vi "nanocal -- nuclear schottky fit -- 2x2 -- V9.vi"() -> ()   [LabVIEW 2021] (continued)
\"στS\" -> 0.003261272874   ,  \"στN\" -> 0.003231373649    |>   , \n\"IDS0512_220604_RAW_cal__sam_\" ->   <|    \"ζ\" -> 0.000000000000   ,  \"τ1\" -> 0.000000000000   ,  \"τS\" -> 0.000000000000   ,  \"τN\" -> 0.000000000000   ,  \"τC\" -> 0.000000000000   ,  \"κ0\" -> 0.000000000000   ,  \"mm1\" -> 0.000000000000   ,  \"mm2\" -> 0.000000000000   ,  \"mm3\" -> 0.000000000000   ,  \"T\" -> 0.250000000000   ,  \"B\" -> 6.000000000000   ,  \"θ\" -> 45.000000000000   ,  \"Reoff\" -> 0.000000000000   ,  \"Imoff\" -> 0.000000000000   ,  \"στ1\" -> 0.000000000000   ,  \"στS\" -> 0.000000000000   ,  \"στN\" -> 0.000000000000    |>   , \n\"IDS0513_220604_RAW_cal__ref_\" ->   <|    \"ζ\" -> 0.109354643265   ,  \"τ1\" -> 0.019745794663   ,  \"τS\" -> 0.045929868636   ,  \"τN\" -> 0.004362632792   ,  \"τC\" -> 0.001089331798   ,  \"κ0\" -> 0.000000001568   ,  \"mm1\" -> 0.000105345441   ,  \"mm2\" -> 0.017323789537   ,  \"mm3\" -> 0.059198211464   ,  \"T\" -> 0.300000000000   ,  \"B\" -> 6.000000000000   ,  \"θ\" -> 45.000000000000   ,  \"Reoff\" -> -9718367.346938773990   ,  \"Imoff\" -> 0.000000000000   ,  \"στ1\" -> 0.000746121350   ,  \"στS\" -> 0.000145078797   ,  \"στN\" -> 0.000139513521    |>   , \n\"IDS0513_220604_RAW_cal__sam_\" ->   <|    \"ζ\" -> 0.000000000000   ,  \"τ1\" -> 0.000000000000   ,  \"τS\" -> 0.000000000000   ,  \"τN\" -> 0.000000000000   ,  \"τC\" -> 0.000000000000   ,  \"κ0\" -> 0.000000000000   ,  \"mm1\" -> 0.000000000000   ,  \"mm2\" -> 0.000000000000   ,  \"mm3\" -> 0.000000000000   ,  \"T\" -> 0.300000000000   ,  \"B\" -> 6.000000000000   ,  \"θ\" -> 45.000000000000   ,  \"Reoff\" -> 0.000000000000   ,  \"Imoff\" -> 0.000000000000   ,  \"στ1\" -> 0.000000000000   ,  \"στS\" -> 0.000000000000   ,  \"στN\" -> 0.000000000000    |>   , \n\"IDS0514_220604_RAW_cal__ref_\" ->   <|    \"ζ\" -> 0.078464971050   ,  \"τ1\" -> 0.017563831776   ,  \"τS\" -> 0.042315631100   ,  \"τN\" -> 0.002449698464   ,  \"τC\" -> 0.001311085354   ,  \"κ0\" -> 0.000000001978   ,  \"mm1\" -> 0.000092908726   ,  \"mm2\" -> 0.016171593309   ,  \"mm3\" -> 0.050888254947   ,  \"T\" -> 0.360000000000   ,  \"B\" -> 6.000000000000   ,  \"θ\" -> 45.000000000000   ,  \"Reoff\" -> -5555102.040816326630   ,  \"Imoff\" -> 0.000000000000   ,  \"στ1\" -> 0.001705710692   ,  \"στS\" -> 0.000224693737   ,  \"στN\" -> 0.000168766252    |>   , \n\"IDS0514_220604_RAW_cal__sam_\" ->   <|    \"ζ\" -> 0.000000000000   ,  \"τ1\" -> 0.000000000000   ,  \"τS\" -> 0.000000000000   ,  \"τN\" -> 0.000000000000   ,  \"τC\" -> 0.000000000000   ,  \"κ0\" -> 0.000000000000   ,  \"mm1\" -> 0.000000000000   ,  \"mm2\" -> 0.000000000000   ,  \"mm3\" -> 0.000000000000   ,  \"T\" -> 0.360000000000   ,  \"B\" -> 6.000000000000   ,  \"θ\" -> 45.000000000000   ,  \"Reoff\" -> 0.000000000000   ,  \"Imoff\" -> 0.000000000000   ,  \"στ1\" -> 0.000000000000   ,  \"στS\" -> 0.000000000000   ,  \"στN\" -> 0.000000000000    |>   , \n\"IDS0515_220604_RAW_cal__ref_\" ->   <|    \"ζ\" -> 0.061585995431   ,  \"τ1\" -> 0.017021907134   ,  \"τS\" -> 0.041190711561   ,  \"τN\" -> 0.001390110365   ,  \"τC\" -> 0.001428995669   ,  \"κ0\" -> 0.000000002390   ,  \"mm1\" -> 0.000080420017   ,  \"mm2\" -> 0.016194561258   ,  \"mm3\" -> 0.047379125758   ,  \"T\" -> 0.430000000000   ,  \"B\" -> 6.000000000000   ,  \"θ\" -> 45.000000000000   ,  \"Reoff\" -> -4253061.224489795980   ,  \"Imoff\" -> 0.000000000000   ,  \"στ1\" -> 0.004152949973   ,  \"στS\" -> 0.000363204682   ,  \"στN\" -> 0.000192260687    |>   , \n\"IDS0515_220604_RAW_cal__sam_\" ->   <|    \"ζ\" -> 0.000000000000   ,  \"τ1\" -> 0.000000000000   ,  \"τS\" -> 0.000000000000   ,  \"τN\" -> 0.000000000000   ,  \"τC\" -> 0.000000000000   ,  \"κ0\" -> 0.000000000000   ,  \"mm1\" -> 0.000000000000   ,  \"mm2\" -> 0.000000000000   ,  \"mm3\" -> 0.000000000000   ,  \"T\" -> 0.430000000000   ,  \"B\" -> 6.000000000000   ,  \"θ\" -> 45.000000000000   ,  \"Reoff\" -> 0.000000000000   ,  \"Imoff\" -> 0.000000000000   ,  \"στ1\" -> 0.000000000000   ,  \"στS\" -> 0.000000000000   ,  \"στN\" -> 0.000000000000    |>   , \n\"IDS0516_220604_RAW_cal__ref_\" ->   <|    \"ζ\" -> 0.045061124228   ,  \"τ1\" -> 0.016174333666   ,  \"τS\" -> 0.041331628225   ,  \"τN\" -> 0.001008746985   ,  \"τC\" -> 0.001666143406   ,  \"κ0\" -> 0.000000003072   ,  \"mm1\" -> 0.000069279556   ,  \"mm2\" -> 0.015610467629   ,  \"mm3\" -> 0.046409010004   ,  \"T\" -> 0.520000000000   ,  \"B\" -> 6.000000000000   ,  \"θ\" -> 45.000000000000   ,  \"Reoff\" -> -2636734.693877550770   ,  \"Imoff\" -> 0.000000000000   ,  \"στ1\" -> 0.000679845630   ,  \"στS\" -> 0.000215440983   ,  \"στN\" -> 0.000036761910    |>   , \n\"IDS0516_220604_RAW_cal__sam_\" ->   <|    \"ζ\" -> 0.000000000000   ,  \"τ1\" -> 0.000000000000   ,  \"τS\" -> 0.000000000000   ,  \"τN\" -> 0.000000000000   ,  \"τC\" -> 0.000000000000   ,  \"κ0\" -> 0.000000000000   ,  \"mm1\" -> 0.000000000000   ,  \"mm2\" -> 0.000000000000   ,  \"mm3\" -> 0.000000000000   ,  \"T\" -> 0.520000000000   ,  \"B\" -> 6.000000000000   ,  \"θ\" -> 45.000000000000   ,  \"Reoff\" -> 0.000000000000   ,  \"Imoff\" -> 0.000000000000   ,  \"στ1\" -> 0.000000000000   ,  \"στS\" -> 0.000000000000   ,  \"στN\" -> 0.000000000000    |>   , \n\"IDS0517_220604_RAW_cal__ref_\" ->   <|    \"ζ\" -> 0.037661249073   ,  \"τ1\" -> 0.016158267438   ,  \"τS\" -> 0.041535470501   ,  \"τN\" -> 0.000589951470   ,  \"τC\" -> 0.001574909889   ,  \"κ0\" -> 0.000000003727   ,  \"mm1\" -> 0.000055213424   ,  \"mm2\" -> 0.015821969361   ,  \"mm3\" -> 0.045567912522   ,  \"T\" -> 0.620000000000   ,  \"B\" -> 6.000000000000   ,  \"θ\" -> 45.000000000000   ,  \"Reoff\" -> -2277551.020408163780   ,  \"Imoff\" -> 0.000000000000   ,  \"στ1\" -> 0.000926762360   ,  \"στS\" -> 0.000192613038   ,  \"στN\" -> 0.000026616394    |>   , \n\"IDS0517_220604_RAW_cal__sam_\" ->   <|    \"ζ\" -> 0.000000000000   ,  \"τ1\" -> 0.000000000000   ,  \"τS\" -> 0.000000000000   ,  \"τN\" -> 0.000000000000   ,  \"τC\" -> 0.000000000000   ,  \"κ0\" -> 0.000000000000   ,  \"mm1\" -> 0.000000000000   ,  \"mm2\" -> 0.000000000000   ,  \"mm3\" -> 0.000000000000   ,  \"T\" -> 0.620000000000   ,  \"B\" -> 6.000000000000   ,  \"θ\" -> 45.000000000000   ,  \"Reoff\" -> 0.000000000000   ,  \"Imoff\" -> 0.000000000000   ,  \"στ1\" -> 0.000000000000   ,  \"στS\" -> 0.000000000000   ,  \"στN\" -> 0.000000000000    |>   , \n\"IDS0518_220604_RAW_cal__ref_\" ->   <|    \"ζ\" -> 0.026897195586   ,  \"τ1\" -> 0.017029322947   ,  \"τS\" -> 0.030300618121   ,  \"τN\" -> 0.000253092893   ,  \"τC\" -> 0.002128020527   ,  \"κ0\" -> 0.000000005137   ,  \"mm1\" -> 0.000052252635   ,  \"mm2\" -> 0.016764147571   ,  \"mm3\" -> 0.033716463424   ,  \"T\" -> 0.820000000000   ,  \"B\" -> 6.000000000000   ,  \"θ\" -> 45.000000000000   ,  \"Reoff\" -> -1020408.163265306500   ,  \"Imoff\" -> 0.000000000000   ,  \"στ1\" -> 0.001120431630   ,  \"στS\" -> 0.000175631796   ,  \"στN\" -> 0.000008557959    |>   , \n\"IDS0518_220604_RAW_cal__sam_\" ->   <|    \"ζ\" -> 0.000000000000   ,  \"τ1\" -> 0.000000000000   ,  \"τS\" -> 0.000000000000   ,  \"τN\" -> 0.000000000000   ,  \"τC\" -> 0.000000000000   ,  \"κ0\" -> 0.000000000000   ,  \"mm1\" -> 0.000000000000   ,  \"mm2\" -> 0.000000000000   ,  \"mm3\" -> 0.000000000000   ,  \"T\" -> 0.820000000000   ,  \"B\" -> 6.000000000000   ,  \"θ\" -> 45.000000000000   ,  \"Reoff\" -> 0.000000000000   ,  \"Imoff\" -> 0.000000000000   ,  \"στ1\" -> 0.000000000000   ,  \"στS\" -> 0.000000000000   ,  \"στN\" -> 0.000000000000    |>   , \n\"IDS0519_220604_RAW_cal__ref_\" ->   <|    \"ζ\" -> 0.022664825895   ,  \"τ1\" -> 0.014721420139   ,  \"τS\" -> 0.018200510248   ,  \"τN\" -> 0.000100851172   ,  \"τC\" -> 0.002380537737   ,  \"κ0\" -> 0.000000007190   ,  \"mm1\" -> 0.000046880798   ,  \"mm2\" -> 0.014490052902   ,  \"mm3\" -> 0.021281182766   ,  \"T\" -> 1.120000000000   ,  \"B\" -> 6.000000000000   ,  \"θ\" -> 45.000000000000   ,  \"Reoff\" -> -795918.367346938698   ,  \"Imoff\" -> 0.000000000000   ,  \"στ1\" -> 0.002006498411   ,  \"στS\" -> 0.000156945460   ,  \"στN\" -> 0.000006591622    |>   , \n\"IDS0519_220604_RAW_cal__sam_\" ->   <|    \"ζ\" -> 0.000000000000   ,  \"τ1\" -> 0.000000000000   ,  \"τS\" -> 0.000000000000   ,  \"τN\" -> 0.000000000000   ,  \"τC\" -> 0.000000000000   ,  \"κ0\" -> 0.000000000000   ,  \"mm1\" -> 0.000000000000   ,  \"mm2\" -> 0.000000000000   ,  \"mm3\" -> 0.000000000000   ,  \"T\" -> 1.120000000000   ,  \"B\" -> 6.000000000000   ,  \"θ\" -> 45.000000000000   ,  \"Reoff\" -> 0.000000000000   ,  \"Imoff\" -> 0.000000000000   ,  \"στ1\" -> 0.000000000000   ,  \"στS\" -> 0.000000000000   ,  \"στN\" -> 0.000000000000    |>   , \n\"IDS0520_220604_RAW_cal__ref_\" ->   <|    \"ζ\" -> 0.017334133227   ,  \"τ1\" -> 0.014742496640   ,  \"τS\" -> 0.012814930706   ,  \"τN\" -> 0.000029321869   ,  \"τC\" -> 0.002644067199   ,  \"κ0\" -> 0.000000012608   ,  \"mm1\" -> 0.000037545170   ,  \"mm2\" -> 0.014397895803   ,  \"mm3\" -> 0.016018019426   ,  \"T\" -> 1.900000000000   ,  \"B\" -> 6.000000000000   ,  \"θ\" -> 45.000000000000   ,  \"Reoff\" -> -346938.775510204955   ,  \"Imoff\" -> 0.000000000000   ,  \"στ1\" -> 0.000944080066   ,  \"στS\" -> 0.000100682155   ,  \"στN\" -> 0.000000473993    |>   , \n\"IDS0520_220604_RAW_cal__sam_\" ->   <|    \"ζ\" -> 0.000000000000   ,  \"τ1\" -> 0.000000000000   ,  \"τS\" -> 0.000000000000   ,  \"τN\" -> 0.000000000000   ,  \"τC\" -> 0.000000000000   ,  \"κ0\" -> 0.000000000000   ,  \"mm1\" -> 0.000000000000   ,  \"mm2\" -> 0.000000000000   ,  \"mm3\" -> 0.000000000000   ,  \"T\" -> 1.900000000000   ,  \"B\" -> 6.000000000000   ,  \"θ\" -> 45.000000000000   ,  \"Reoff\" -> 0.000000000000   ,  \"Imoff\" -> 0.000000000000   ,  \"στ1\" -> 0.000000000000   ,  \"στS\" -> 0.000000000000   ,  \"στN\" -> 0.000000000000    |>   , \n\"IDS0521_220604_RAW_cal__ref_\" ->   <|    \"ζ\" -> 0.016488778700   ,  \"τ1\" -> 0.014739187925   ,  \"τS\" -> 0.009276506923   ,  \"τN\" -> 0.000009013062   ,  \"τC\" -> 0.002584186338   ,  \"κ0\" -> 0.000000022490   ,  \"mm1\" -> 0.000032992550   ,  \"mm2\" -> 0.011941581665   ,  \"mm3\" -> 0.014787426917   ,  \"T\" -> 3.100000000000   ,  \"B\" -> 6.000000000000   ,  \"θ\" -> 45.000000000000   ,  \"Reoff\" -> -167346.938775509596   ,  \"Imoff\" -> 0.000000000000   ,  \"στ1\" -> 0.000306328571   ,  \"στS\" -> 0.000088607277   ,  \"στN\" -> 0.000000155207    |>   , \n\"IDS0521_220604_RAW_cal__sam_\" ->   <|    \"ζ\" -> 0.000000000000   ,  \"τ1\" -> 0.000000000000   ,  \"τS\" -> 0.000000000000   ,  \"τN\" -> 0.000000000000   ,  \"τC\" -> 0.000000000000   ,  \"κ0\" -> 0.000000000000   ,  \"mm1\" -> 0.000000000000   ,  \"mm2\" -> 0.000000000000   ,  \"mm3\" -> 0.000000000000   ,  \"T\" -> 3.100000000000   ,  \"B\" -> 6.000000000000   ,  \"θ\" -> 45.000000000000   ,  \"Reoff\" -> 0.000000000000   ,  \"Imoff\" -> 0.000000000000   ,  \"στ1\" -> 0.000000000000   ,  \"στS\" -> 0.000000000000   ,  \"στN\" -> 0.000000000000    |>   , \n\"IDS0523_220604_RAW_cal__ref_\" ->   <|    \"ζ\" -> 0.248494287035   ,  \"τ1\" -> 0.140471463831   ,  \"τS\" -> 0.029170563772   ,  \"τN\" -> 0.016077523258   ,  \"τC\" -> 0.000858124054   ,  \"κ0\" -> 0.000000000897   ,  \"mm1\" -> 0.000167616779   ,  \"mm2\" -> 0.031344824749   ,  \"mm3\" -> 0.166309124513   ,  \"T\" -> 0.200000000000   ,  \"B\" -> 4.000000000000   ,  \"θ\" -> 45.000000000000   ,  \"Reoff\" -> -41942857.142857194000   ,  \"Imoff\" -> 0.000000000000   ,  \"στ1\" -> 0.163113161678   ,  \"στS\" -> 0.000492211177   ,  \"στN\" -> 0.015881366148    |>   , \n\"IDS0523_220604_RAW_cal__sam_\" ->   <|    \"ζ\" -> 0.000000000000   ,  \"τ1\" -> 0.000000000000   ,  \"τS\" -> 0.000000000000   ,  \"τN\" -> 0.000000000000   ,  \"τC\" -> 0.000000000000   ,  \"κ0\" -> 0.000000000000   ,  \"mm1\" -> 0.000000000000   ,  \"mm2\" -> 0.000000000000   ,  \"mm3\" -> 0.000000000000   ,  \"T\" -> 0.200000000000   ,  \"B\" -> 4.000000000000   ,  \"θ\" -> 45.000000000000   ,  \"Reoff\" -> 0.000000000000   ,  \"Imoff\" -> 0.000000000000   ,  \"στ1\" -> 0.000000000000   ,  \"στS\" -> 0.000000000000   ,  \"στN\" -> 0.000000000000    |>   , \n\"IDS0524_220605_RAW_cal__ref_\" ->   <|    \"ζ\" -> 0.342264426031   ,  \"τ1\" -> 0.148951865550   ,  \"τS\" -> 0.034223286872   ,  \"τN\" -> 0.023114154081   ,  \"τC\" -> 0.000835537193   ,  \"κ0\" -> 0.000000000715   ,  \"mm1\" -> 0.000210189792   ,  \"mm2\" -> 0.036494538053   ,  \"mm3\" -> 0.190044682168   ,  \"T\" -> 0.170000000000   ,  \"B\" -> 4.000000000000   ,  \"θ\" -> 45.000000000000   ,  \"Reoff\" -> -68526530.612244904100   ,  \"Imoff\" -> 0.000000000000   ,  \"στ1\" -> 0.142355896146   ,  \"στS\" -> 0.002021018584   ,  \"στN\" -> 0.017181504971    |>   , \n\"IDS0524_220605_RAW_cal__sam_\" ->   <|    \"ζ\" -> 0.000000000000   ,  \"τ1\" -> 0.000000000000   ,  \"τS\" -> 0.000000000000   ,  \"τN\" -> 0.000000000000   ,  \"τC\" -> 0.000000000000   ,  \"κ0\" -> 0.000000000000   ,  \"mm1\" -> 0.000000000000   ,  \"mm2\" -> 0.000000000000   ,  \"mm3\" -> 0.000000000000   ,  \"T\" -> 0.170000000000   ,  \"B\" -> 4.000000000000   ,  \"θ\" -> 45.000000000000   ,  \"Reoff\" -> 0.000000000000   ,  \"Imoff\" -> 0.000000000000   ,  \"στ1\" -> 0.000000000000   ,  \"στS\" -> 0.000000000000   ,  \"στN\" -> 0.000000000000    |>   , \n\"IDS0525_220605_RAW_cal__ref_\" ->   <|    \"ζ\" -> 0.438280595131   ,  \"τ1\" -> 0.137342772879   ,  \"τS\" -> 0.040264580872   ,  \"τN\" -> 0.033372414925   ,  \"τC\" -> 0.000857425660   ,  \"κ0\" -> 0.000000000589   ,  \"mm1\" -> 0.000258601158   ,  \"mm2\" -> 0.039283249404   ,  \"mm3\" -> 0.204569010116   ,  \"T\" -> 0.150000000000   ,  \"B\" -> 4.000000000000   ,  \"θ\" -> 45.000000000000   ,  \"Reoff\" -> -86930612.244897961600   ,  \"Imoff\" -> 0.000000000000   ,  \"στ1\" -> 0.199442289109   ,  \"στS\" -> 0.005269413629   ,  \"στN\" -> 0.036619051524    |>   , \n\"IDS0525_220605_RAW_cal__sam_\" ->   <|    \"ζ\" -> 0.000000000000   ,  \"τ1\" -> 0.000000000000   ,  \"τS\" -> 0.000000000000   ,  \"τN\" -> 0.000000000000   ,  \"τC\" -> 0.000000000000   ,  \"κ0\" -> 0.000000000000   ,  \"mm1\" -> 0.000000000000   ,  \"mm2\" -> 0.000000000000   ,  \"mm3\" -> 0.000000000000   ,  \"T\" -> 0.150000000000   ,  \"B\" -> 4.000000000000   ,  \"θ\" -> 45.000000000000   ,  \"Reoff\" -> 0.000000000000   ,  \"Imoff\" -> 0.000000000000   ,  \"στ1\" -> 0.000000000000   ,  \"στS\" -> 0.000000000000   ,  \"στN\" -> 0.000000000000    |>   , \n\"IDS0526_220605_RAW_cal__ref_\" ->   <|    \"ζ\" -> 0.681535842582   ,  \"τ1\" -> 0.096440830636   ,  \"τS\" -> 0.049346041453   ,  \"τN\" -> 0.056139024949   ,  \"τC\" -> 0.000822867948   ,  \"κ0\" -> 0.000000000444   ,  \"mm1\" -> 0.000331542094   ,  \"mm2\" -> 0.033417308945   ,  \"mm3\" -> 0.240891767557   ,  \"T\" -> 0.120000000000   ,  \"B\" -> 4.000000000000   ,  \"θ\" -> 45.000000000000   ,  \"Reoff\" -> -183040816.326530635000   ,  \"Imoff\" -> 0.000000000000   ,  \"στ1\" -> 0.106020317496   ,  \"στS\" -> 0.010756317478   ,  \"στN\" -> 0.041433473525    |>   , \n\"IDS0526_220605_RAW_cal__sam_\" ->   <|    \"ζ\" -> 0.000000000000   ,  \"τ1\" -> 0.000000000000   ,  \"τS\" -> 0.000000000000   ,  \"τN\" -> 0.000000000000   ,  \"τC\" -> 0.000000000000   ,  \"κ0\" -> 0.000000000000   ,  \"mm1\" -> 0.000000000000   ,  \"mm2\" -> 0.000000000000   ,  \"mm3\" -> 0.000000000000   ,  \"T\" -> 0.120000000000   ,  \"B\" -> 4.000000000000   ,  \"θ\" -> 45.000000000000   ,  \"Reoff\" -> 0.000000000000   ,  \"Imoff\" -> 0.000000000000   ,  \"στ1\" -> 0.000000000000   ,  \"στS\" -> 0.000000000000   ,  \"στN\" -> 0.000000000000    |>   , \n\"IDS0527_220605_RAW_cal__ref_\" ->   <|    \"ζ\" -> 0.163587274330   ,  \"τ1\" -> 0.177723598175   ,  \"τS\" -> 0.024747362505   ,  \"τN\" -> 0.010499593471   ,  \"τC\" -> 0.000964995814   ,  \"κ0\" -> 0.000000001207   ,  \"mm1\" -> 0.000131851499   ,  \"mm2\" -> 0.027402099160   ,  \"mm3\" -> 0.192167552763   ,  \"T\" -> 0.250000000000   ,  \"B\" -> 4.000000000000   ,  \"θ\" -> 45.000000000000   ,  \"Reoff\" -> -21493877.551020443400   ,  \"Imoff\" -> 0.000000000000   ,  \"στ1\" -> 0.096620218228   ,  \"στS\" -> 0.000434999932   ,  \"στN\" -> 0.007322093866    |>   , \n\"IDS0527_220605_RAW_cal__sam_\" ->   <|    \"ζ\" -> 0.000000000000   ,  \"τ1\" -> 0.000000000000   ,  \"τS\" -> 0.000000000000   ,  \"τN\" -> 0.000000000000   ,  \"τC\" -> 0.000000000000   ,  \"κ0\" -> 0.000000000000   ,  \"mm1\" -> 0.000000000000   ,  \"mm2\" -> 0.000000000000   ,  \"mm3\" -> 0.000000000000   ,  \"T\" -> 0.250000000000   ,  \"B\" -> 4.000000000000   ,  \"θ\" -> 45.000000000000   ,  \"Reoff\" -> 0.000000000000   ,  \"Imoff\" -> 0.000000000000   ,  \"στ1\" -> 0.000000000000   ,  \"στS\" -> 0.000000000000   ,  \"στN\" -> 0.000000000000    |>   , \n\"IDS0528_220605_RAW_cal__ref_\" ->   <|    \"ζ\" -> 0.115342924881   ,  \"τ1\" -> 0.183028972039   ,  \"τS\" -> 0.022615118092   ,  \"τN\" -> 0.006941794186   ,  \"τC\" -> 0.001037906865   ,  \"κ0\" -> 0.000000001545   ,  \"mm1\" -> 0.000103500075   ,  \"mm2\" -> 0.024936932480   ,  \"mm3\" -> 0.191992539340   ,  \"T\" -> 0.300000000000   ,  \"B\" -> 4.000000000000   ,  \"θ\" -> 45.000000000000   ,  \"Reoff\" -> -13363265.306122444600   ,  \"Imoff\" -> 0.000000000000   ,  \"στ1\" -> 0.063499413801   ,  \"στS\" -> 0.000291757985   ,  \"στN\" -> 0.002527808179    |>   , \n\"IDS0528_220605_RAW_cal__sam_\" ->   <|    \"ζ\" -> 0.000000000000   ,  \"τ1\" -> 0.000000000000   ,  \"τS\" -> 0.000000000000   ,  \"τN\" -> 0.000000000000   ,  \"τC\" -> 0.000000000000   ,  \"κ0\" -> 0.000000000000   ,  \"mm1\" -> 0.000000000000   ,  \"mm2\" -> 0.000000000000   ,  \"mm3\" -> 0.000000000000   ,  \"T\" -> 0.300000000000   ,  \"B\" -> 4.000000000000   ,  \"θ\" -> 45.000000000000   ,  \"Reoff\" -> 0.000000000000   ,  \"Imoff\" -> 0.000000000000   ,  \"στ1\" -> 0.000000000000   ,  \"στS\" -> 0.000000000000   ,  \"στN\" -> 0.000000000000    |>   , \n\"IDS0529_220605_RAW_cal__ref_\" ->   <|    \"ζ\" -> 0.082205302754   ,  \"τ1\" -> 0.199068291340   ,  \"τS\" -> 0.021395603563   ,  \"τN\" -> 0.004747138238   ,  \"τC\" -> 0.001295613399   ,  \"κ0\" -> 0.000000001948   ,  \"mm1\" -> 0.000093558415   ,  \"mm2\" -> 0.023663557896   ,  \"mm3\" -> 0.204898602234   ,  \"T\" -> 0.360000000000   ,  \"B\" -> 4.000000000000   ,  \"θ\" -> 45.000000000000   ,  \"Reoff\" -> -6702040.816326528790   ,  \"Imoff\" -> 0.000000000000   ,  \"στ1\" -> 0.038070369381   ,  \"στS\" -> 0.000151057018   ,  \"στN\" -> 0.001245904687    |>   , \n\"IDS0529_220605_RAW_cal__sam_\" ->   <|    \"ζ\" -> 0.000000000000   ,  \"τ1\" -> 0.000000000000   ,  \"τS\" -> 0.000000000000   ,  \"τN\" -> 0.000000000000   ,  \"τC\" -> 0.000000000000   ,  \"κ0\" -> 0.000000000000   ,  \"mm1\" -> 0.000000000000   ,  \"mm2\" -> 0.000000000000   ,  \"mm3\" -> 0.000000000000   ,  \"T\" -> 0.360000000000   ,  \"B\" -> 4.000000000000   ,  \"θ\" -> 45.000000000000   ,  \"Reoff\" -> 0.000000000000   ,  \"Imoff\" -> 0.000000000000   ,  \"στ1\" -> 0.000000000000   ,  \"στS\" -> 0.000000000000   ,  \"στN\" -> 0.000000000000    |>   , \n\"IDS0530_220605_RAW_cal__ref_\" ->   <|    \"ζ\" -> 0.062434773086   ,  \"τ1\" -> 0.091033034747   ,  \"τS\" -> 0.021000801063   ,  \"τN\" -> 0.002166413652   ,  \"τC\" -> 0.001607646673   ,  \"κ0\" -> 0.000000002334   ,  \"mm1\" -> 0.000088451406   ,  \"mm2\" -> 0.023050943702   ,  \"mm3\" -> 0.094114940821   ,  \"T\" -> 0.420000000000   ,  \"B\" -> 4.000000000000   ,  \"θ\" -> 45.000000000000   ,  \"Reoff\" -> -3579591.836734689770   ,  \"Imoff\" -> 0.000000000000   ,  \"στ1\" -> 0.001625101640   ,  \"στS\" -> 0.000103039832   ,  \"στN\" -> 0.000006624579    |>   , \n\"IDS0530_220605_RAW_cal__sam_\" ->   <|    \"ζ\" -> 0.000000000000   ,  \"τ1\" -> 0.000000000000   ,  \"τS\" -> 0.000000000000   ,  \"τN\" -> 0.000000000000   ,  \"τC\" -> 0.000000000000   ,  \"κ0\" -> 0.000000000000   ,  \"mm1\" -> 0.000000000000   ,  \"mm2\" -> 0.000000000000   ,  \"mm3\" -> 0.000000000000   ,  \"T\" -> 0.420000000000   ,  \"B\" -> 4.000000000000   ,  \"θ\" -> 45.000000000000   ,  \"Reoff\" -> 0.000000000000   ,  \"Imoff\" -> 0.000000000000   ,  \"στ1\" -> 0.000000000000   ,  \"στS\" -> 0.000000000000   ,  \"στN\" -> 0.000000000000    |>   , \n\"IDS0531_220605_RAW_cal__ref_\" ->   <|    \"ζ\" -> 0.047292360430   ,  \"τ1\" -> 0.215650832524   ,  \"τS\" -> 0.021748628873   ,  \"τN\" -> 0.002014257649   ,  \"τC\" -> 0.001656178311   ,  \"κ0\" -> 0.000000003034   ,  \"mm1\" -> 0.000069918264   ,  \"mm2\" -> 0.024098100915   ,  \"mm3\" -> 0.218025681173   ,  \"T\" -> 0.520000000000   ,  \"B\" -> 4.000000000000   ,  \"θ\" -> 45.000000000000   ,  \"Reoff\" -> -2955102.040816321970   ,  \"Imoff\" -> 0.000000000000   ,  \"στ1\" -> 0.046963197390   ,  \"στS\" -> 0.000145543572   ,  \"στN\" -> 0.000181922698    |>   , \n\"IDS0531_220605_RAW_cal__sam_\" ->   <|    \"ζ\" -> 0.000000000000   ,  \"τ1\" -> 0.000000000000   ,  \"τS\" -> 0.000000000000   ,  \"τN\" -> 0.000000000000   ,  \"τC\" -> 0.000000000000   ,  \"κ0\" -> 0.000000000000   ,  \"mm1\" -> 0.000000000000   ,  \"mm2\" -> 0.000000000000   ,  \"mm3\" -> 0.000000000000   ,  \"T\" -> 0.520000000000   ,  \"B\" -> 4.000000000000   ,  \"θ\" -> 45.000000000000   ,  \"Reoff\" -> 0.000000000000   ,  \"Imoff\" -> 0.000000000000   ,  \"στ1\" -> 0.000000000000   ,  \"στS\" -> 0.000000000000   ,  \"στN\" -> 0.000000000000    |>   , \n\"IDS0532_220605_RAW_cal__ref_\" ->   <|    \"ζ\" -> 0.039581980273   ,  \"τ1\" -> 0.217269361754   ,  \"τS\" -> 0.023071327438   ,  \"τN\" -> 0.001182618434   ,  \"τC\" -> 0.001652851775   ,  \"κ0\" -> 0.000000003717   ,  \"mm1\" -> 0.000059010683   ,  \"mm2\" -> 0.025415535832   ,  \"mm3\" -> 0.218661632092   ,  \"T\" -> 0.620000000000   ,  \"B\" -> 4.000000000000   ,  \"θ\" -> 45.000000000000   ,  \"Reoff\" -> -2746938.775510199370   ,  \"Imoff\" -> 0.000000000000   ,  \"στ1\" -> 0.015098698436   ,  \"στS\" -> 0.000189797573   ,  \"στN\" -> 0.000008998512    |>   , \n\"IDS0532_220605_RAW_cal__sam_\" ->   <|    \"ζ\" -> 0.000000000000   ,  \"τ1\" -> 0.000000000000   ,  \"τS\" -> 0.000000000000   ,  \"τN\" -> 0.000000000000   ,  \"τC\" -> 0.000000000000   ,  \"κ0\" -> 0.000000000000   ,  \"mm1\" -> 0.000000000000   ,  \"mm2\" -> 0.000000000000   ,  \"mm3\" -> 0.000000000000   ,  \"T\" -> 0.620000000000   ,  \"B\" -> 4.000000000000   ,  \"θ\" -> 45.000000000000   ,  \"Reoff\" -> 0.000000000000   ,  \"Imoff\" -> 0.000000000000   ,  \"στ1\" -> 0.000000000000   ,  \"στS\" -> 0.000000000000   ,  \"στN\" -> 0.000000000000    |>   , \n\"IDS0533_220605_RAW_cal__ref_\" ->   <|    \"ζ\" -> 0.026006399704   ,  \"τ1\" -> 0.219491604326   ,  \"τS\" -> 0.026508960211   ,  \"τN\" -> 0.000691251356   ,  \"τC\" -> 0.002192117759   ,  \"κ0\" -> 0.000000005099   ,  \"mm1\" -> 0.000051510023   ,  \"mm2\" -> 0.029230026409   ,  \"mm3\" -> 0.220309776794   ,  \"T\" -> 0.820000000000   ,  \"B\" -> 4.000000000000   ,  \"θ\" -> 45.000000000000   ,  \"Reoff\" -> -873469.387755103408   ,  \"Imoff\" -> 0.000000000000   ,  \"στ1\" -> 0.040897544111   ,  \"στS\" -> 0.000189265066   ,  \"στN\" -> 0.000022111002    |>   , \n\"IDS0533_220605_RAW_cal__sam_\" ->   <|    \"ζ\" -> 0.000000000000   ,  \"τ1\" -> 0.000000000000   ,  \"τS\" -> 0.000000000000   ,  \"τN\" -> 0.000000000000   ,  \"τC\" -> 0.000000000000   ,  \"κ0\" -> 0.000000000000   ,  \"mm1\" -> 0.000000000000   ,  \"mm2\" -> 0.000000000000   ,  \"mm3\" -> 0.000000000000   ,  \"T\" -> 0.820000000000   ,  \"B\" -> 4.000000000000   ,  \"θ\" -> 45.000000000000   ,  \"Reoff\" -> 0.000000000000   ,  \"Imoff\" -> 0.000000000000   ,  \"στ1\" -> 0.000000000000   ,  \"στS\" -> 0.000000000000   ,  \"στN\" -> 0.000000000000    |>   , \n\"IDS0534_220605_RAW_cal__ref_\" ->   <|    \"ζ\" -> 0.022451049934   ,  \"τ1\" -> 0.221358754558   ,  \"τS\" -> 0.033966694492   ,  \"τN\" -> 0.000363309481   ,  \"τC\" -> 0.002245679298   ,  \"κ0\" -> 0.000000007138   ,  \"mm1\" -> 0.000046374039   ,  \"mm2\" -> 0.036854393963   ,  \"mm3\" -> 0.221804414461   ,  \"T\" -> 1.120000000000   ,  \"B\" -> 4.000000000000   ,  \"θ\" -> 45.000000000000   ,  \"Reoff\" -> -885714.285714285447   ,  \"Imoff\" -> 0.000000000000   ,  \"στ1\" -> 0.023144908767   ,  \"στS\" -> 0.000217300505   ,  \"στN\" -> 0.000007634517    |>   , \n\"IDS0534_220605_RAW_cal__sam_\" ->   <|    \"ζ\" -> 0.000000000000   ,  \"τ1\" -> 0.000000000000   ,  \"τS\" -> 0.000000000000   ,  \"τN\" -> 0.000000000000   ,  \"τC\" -> 0.000000000000   ,  \"κ0\" -> 0.000000000000   ,  \"mm1\" -> 0.000000000000   ,  \"mm2\" -> 0.000000000000   ,  \"mm3\" -> 0.000000000000   ,  \"T\" -> 1.120000000000   ,  \"B\" -> 4.000000000000   ,  \"θ\" -> 45.000000000000   ,  \"Reoff\" -> 0.000000000000   ,  \"Imoff\" -> 0.000000000000   ,  \"στ1\" -> 0.000000000000   ,  \"στS\" -> 0.000000000000   ,  \"στN\" -> 0.000000000000    |>   , \n\"IDS0535_220605_RAW_cal__ref_\" ->   <|    \"ζ\" -> 0.019576865757   ,  \"τ1\" -> 0.218088277374   ,  \"τS\" -> 0.022473990539   ,  \"τN\" -> 0.000172254737   ,  \"τC\" -> 0.002442141955   ,  \"κ0\" -> 0.000000011417   ,  \"mm1\" -> 0.000042446249   ,  \"mm2\" -> 0.025290622371   ,  \"mm3\" -> 0.218286938488   ,  \"T\" -> 1.700000000000   ,  \"B\" -> 4.000000000000   ,  \"θ\" -> 45.000000000000   ,  \"Reoff\" -> -322448.979591836221   ,  \"Imoff\" -> 0.000000000000   ,  \"στ1\" -> 0.063627358635   ,  \"στS\" -> 0.000720787697   ,  \"στN\" -> 0.000014224220    |>   , \n\"IDS0535_220605_RAW_cal__sam_\" ->   <|    \"ζ\" -> 0.000000000000   ,  \"τ1\" -> 0.000000000000   ,  \"τS\" -> 0.000000000000   ,  \"τN\" -> 0.000000000000   ,  \"τC\" -> 0.000000000000   ,  \"κ0\" -> 0.000000000000   ,  \"mm1\" -> 0.000000000000   ,  \"mm2\" -> 0.000000000000   ,  \"mm3\" -> 0.000000000000   ,  \"T\" -> 1.700000000000   ,  \"B\" -> 4.000000000000   ,  \"θ\" -> 45.000000000000   ,  \"Reoff\" -> 0.000000000000   ,  \"Imoff\" -> 0.000000000000   ,  \"στ1\" -> 0.000000000000   ,  \"στS\" -> 0.000000000000   ,  \"στN\" -> 0.000000000000    |>   , \n\"IDS0536_220605_RAW_cal__ref_\" ->   <|    \"ζ\" -> 0.017203827920   ,  \"τ1\" -> 0.213925239716   ,  \"τS\" -> 0.013557235716   ,  \"τN\" -> 0.000118116880   ,  \"τC\" -> 0.002620828700   ,  \"κ0\" -> 0.000000012687   ,  \"mm1\" -> 0.000037331962   ,  \"mm2\" -> 0.016364021106   ,  \"mm3\" -> 0.214055336357   ,  \"T\" -> 1.900000000000   ,  \"B\" -> 4.000000000000   ,  \"θ\" -> 45.000000000000   ,  \"Reoff\" -> -322448.979591836221   ,  \"Imoff\" -> 0.000000000000   ,  \"στ1\" -> 0.007920167579   ,  \"στS\" -> 0.000110474044   ,  \"στN\" -> 0.000002075732    |>   , \n\"IDS0536_220605_RAW_cal__sam_\" ->   <|    \"ζ\" -> 0.000000000000   ,  \"τ1\" -> 0.000000000000   ,  \"τS\" -> 0.000000000000   ,  \"τN\" -> 0.000000000000   ,  \"τC\" -> 0.000000000000   ,  \"κ0\" -> 0.000000000000   ,  \"mm1\" -> 0.000000000000   ,  \"mm2\" -> 0.000000000000   ,  \"mm3\" -> 0.000000000000   ,  \"T\" -> 1.900000000000   ,  \"B\" -> 4.000000000000   ,  \"θ\" -> 45.000000000000   ,  \"Reoff\" -> 0.000000000000   ,  \"Imoff\" -> 0.000000000000   ,  \"στ1\" -> 0.000000000000   ,  \"στS\" -> 0.000000000000   ,  \"στN\" -> 0.000000000000    |>   , \n\"IDS0537_220605_RAW_cal__ref_\" ->   <|    \"ζ\" -> 0.016837588937   ,  \"τ1\" -> 0.214083726987   ,  \"τS\" -> 0.009462256875   ,  \"τN\" -> 0.000044961797   ,  \"τC\" -> 0.002520072033   ,  \"κ0\" -> 0.000000022492   ,  \"mm1\" -> 0.000033158698   ,  \"mm2\" -> 0.012105753537   ,  \"mm3\" -> 0.214132184097   ,  \"T\" -> 3.100000000000   ,  \"B\" -> 4.000000000000   ,  \"θ\" -> 45.000000000000   ,  \"Reoff\" -> -200000.000000000000   ,  \"Imoff\" -> 0.000000000000   ,  \"στ1\" -> 0.041355363203   ,  \"στS\" -> 0.000204828997   ,  \"στN\" -> 0.000003281967    |>   , \n\"IDS0537_220605_RAW_cal__sam_\" ->   <|    \"ζ\" -> 0.000000000000   ,  \"τ1\" -> 0.000000000000   ,  \"τS\" -> 0.000000000000   ,  \"τN\" -> 0.000000000000   ,  \"τC\" -> 0.000000000000   ,  \"κ0\" -> 0.000000000000   ,  \"mm1\" -> 0.000000000000   ,  \"mm2\" -> 0.000000000000   ,  \"mm3\" -> 0.000000000000   ,  \"T\" -> 3.100000000000   ,  \"B\" -> 4.000000000000   ,  \"θ\" -> 45.000000000000   ,  \"Reoff\" -> 0.000000000000   ,  \"Imoff\" -> 0.000000000000   ,  \"στ1\" -> 0.000000000000   ,  \"στS\" -> 0.000000000000   ,  \"στN\" -> 0.000000000000    |>   , \n\"IDS0538_220605_RAW_cal__ref_\" ->   <|    \"ζ\" -> 0.019986975905   ,  \"τ1\" -> 0.213955272188   ,  \"τS\" -> 0.005937059985   ,  \"τN\" -> 0.000017131866   ,  \"τC\" -> 0.001979607590   ,  \"κ0\" -> 0.000000055230   ,  \"mm1\" -> 0.000029341516   ,  \"mm2\" -> 0.008005311507   ,  \"mm3\" -> 0.213973424895   ,  \"T\" -> 5.700000000000   ,  \"B\" -> 4.000000000000   ,  \"θ\" -> 45.000000000000   ,  \"Reoff\" -> -77551.020408162847   ,  \"Imoff\" -> 0.000000000000   ,  \"στ1\" -> 0.013237190857   ,  \"στS\" -> 0.000032983186   ,  \"στN\" -> 0.000000229969    |>   , \n\"IDS0538_220605_RAW_cal__sam_\" ->   <|    \"ζ\" -> 0.000000000000   ,  \"τ1\" -> 0.000000000000   ,  \"τS\" -> 0.000000000000   ,  \"τN\" -> 0.000000000000   ,  \"τC\" -> 0.000000000000   ,  \"κ0\" -> 0.000000000000   ,  \"mm1\" -> 0.000000000000   ,  \"mm2\" -> 0.000000000000   ,  \"mm3\" -> 0.000000000000   ,  \"T\" -> 5.700000000000   ,  \"B\" -> 4.000000000000   ,  \"θ\" -> 45.000000000000   ,  \"Reoff\" -> 0.000000000000   ,  \"Imoff\" -> 0.000000000000   ,  \"στ1\" -> 0.000000000000   ,  \"στS\" -> 0.000000000000   ,  \"στN\" -> 0.000000000000    |>   , \n\"IDS0540_220605_RAW_cal__ref_\" ->   <|    \"ζ\" -> 0.251392330354   ,  \"τ1\" -> 0.346377607558   ,  \"τS\" -> 0.016513842206   ,  \"τN\" -> 0.014262469720   ,  \"τC\" -> 0.000857308117   ,  \"κ0\" -> 0.000000000886   ,  \"mm1\" -> 0.000166652692   ,  \"mm2\" -> 0.020248144591   ,  \"mm3\" -> 0.365333359092   ,  \"T\" -> 0.200000000000   ,  \"B\" -> 2.000000000000   ,  \"θ\" -> 45.000000000000   ,  \"Reoff\" -> -46204081.632653057600   ,  \"Imoff\" -> 0.000000000000   ,  \"στ1\" -> 0.424749382693   ,  \"στS\" -> 0.000332071104   ,  \"στN\" -> 0.013507044944    |>   , \n\"IDS0540_220605_RAW_cal__sam_\" ->   <|    \"ζ\" -> 0.000000000000   ,  \"τ1\" -> 0.000000000000   ,  \"τS\" -> 0.000000000000   ,  \"τN\" -> 0.000000000000   ,  \"τC\" -> 0.000000000000   ,  \"κ0\" -> 0.000000000000   ,  \"mm1\" -> 0.000000000000   ,  \"mm2\" -> 0.000000000000   ,  \"mm3\" -> 0.000000000000   ,  \"T\" -> 0.200000000000   ,  \"B\" -> 2.000000000000   ,  \"θ\" -> 45.000000000000   ,  \"Reoff\" -> 0.000000000000   ,  \"Imoff\" -> 0.000000000000   ,  \"στ1\" -> 0.000000000000   ,  \"στS\" -> 0.000000000000   ,  \"στN\" -> 0.000000000000    |>   , \n\"IDS0541_220605_RAW_cal__ref_\" ->   <|    \"ζ\" -> 0.165113897347   ,  \"τ1\" -> 0.387980452993   ,  \"τS\" -> 0.014374929410   ,  \"τN\" -> 0.009383556190   ,  \"τC\" -> 0.000942269686   ,  \"κ0\" -> 0.000000001199   ,  \"mm1\" -> 0.000127336399   ,  \"mm2\" -> 0.017060680127   ,  \"mm3\" -> 0.399416047906   ,  \"T\" -> 0.250000000000   ,  \"B\" -> 2.000000000000   ,  \"θ\" -> 45.000000000000   ,  \"Reoff\" -> -23306122.448979616200   ,  \"Imoff\" -> 0.000000000000   ,  \"στ1\" -> 0.067668625614   ,  \"στS\" -> 0.000112915267   ,  \"στN\" -> 0.002227405906    |>   , \n\"IDS0541_220605_RAW_cal__sam_\" ->   <|    \"ζ\" -> 0.000000000000   ,  \"τ1\" -> 0.000000000000   ,  \"τS\" -> 0.000000000000   ,  \"τN\" -> 0.000000000000   ,  \"τC\" -> 0.000000000000   ,  \"κ0\" -> 0.000000000000   ,  \"mm1\" -> 0.000000000000   ,  \"mm2\" -> 0.000000000000   ,  \"mm3\" -> 0.000000000000   ,  \"T\" -> 0.250000000000   ,  \"B\" -> 2.000000000000   ,  \"θ\" -> 45.000000000000   ,  \"Reoff\" -> 0.000000000000   ,  \"Imoff\" -> 0.000000000000   ,  \"στ1\" -> 0.000000000000   ,  \"στS\" -> 0.000000000000   ,  \"στN\" -> 0.000000000000    |>   , \n\"IDS0542_220606_RAW_cal__ref_\" ->   <|    \"ζ\" -> 0.345710784026   ,  \"τ1\" -> 0.327857477320   ,  \"τS\" -> 0.019203362427   ,  \"τN\" -> 0.016889536551   ,  \"τC\" -> 0.000830598267   ,  \"κ0\" -> 0.000000000695   ,  \"mm1\" -> 0.000208359489   ,  \"mm2\" -> 0.024619495516   ,  \"mm3\" -> 0.352430823963   ,  \"T\" -> 0.170000000000   ,  \"B\" -> 2.000000000000   ,  \"θ\" -> 45.000000000000   ,  \"Reoff\" -> -73265306.122448980800   ,  \"Imoff\" -> 0.000000000000   ,  \"στ1\" -> 0.369953882310   ,  \"στS\" -> 0.000610690630   ,  \"στN\" -> 0.016945730597    |>   , \n\"IDS0542_220606_RAW_cal__sam_\" ->   <|    \"ζ\" -> 0.000000000000   ,  \"τ1\" -> 0.000000000000   ,  \"τS\" -> 0.000000000000   ,  \"τN\" -> 0.000000000000   ,  \"τC\" -> 0.000000000000   ,  \"κ0\" -> 0.000000000000   ,  \"mm1\" -> 0.000000000000   ,  \"mm2\" -> 0.000000000000   ,  \"mm3\" -> 0.000000000000   ,  \"T\" -> 0.170000000000   ,  \"B\" -> 2.000000000000   ,  \"θ\" -> 45.000000000000   ,  \"Reoff\" -> 0.000000000000   ,  \"Imoff\" -> 0.000000000000   ,  \"στ1\" -> 0.000000000000   ,  \"στS\" -> 0.000000000000   ,  \"στN\" -> 0.000000000000    |>   , \n\"IDS0543_220606_RAW_cal__ref_\" ->   <|    \"ζ\" -> 0.443467990428   ,  \"τ1\" -> 0.317886288494   ,  \"τS\" -> 0.021647161508   ,  \"τN\" -> 0.018036346988   ,  \"τC\" -> 0.000838651939   ,  \"κ0\" -> 0.000000000590   ,  \"mm1\" -> 0.000252909908   ,  \"mm2\" -> 0.029199801325   ,  \"mm3\" -> 0.346554103461   ,  \"T\" -> 0.150000000000   ,  \"B\" -> 2.000000000000   ,  \"θ\" -> 45.000000000000   ,  \"Reoff\" -> -94081632.653061270700   ,  \"Imoff\" -> 0.000000000000   ,  \"στ1\" -> 0.633667064980   ,  \"στS\" -> 0.001327852543   ,  \"στN\" -> 0.033112841100    |>   , \n\"IDS0543_220606_RAW_cal__sam_\" ->   <|    \"ζ\" -> 0.000000000000   ,  \"τ1\" -> 0.000000000000   ,  \"τS\" -> 0.000000000000   ,  \"τN\" -> 0.000000000000   ,  \"τC\" -> 0.000000000000   ,  \"κ0\" -> 0.000000000000   ,  \"mm1\" -> 0.000000000000   ,  \"mm2\" -> 0.000000000000   ,  \"mm3\" -> 0.000000000000   ,  \"T\" -> 0.150000000000   ,  \"B\" -> 2.000000000000   ,  \"θ\" -> 45.000000000000   ,  \"Reoff\" -> 0.000000000000   ,  \"Imoff\" -> 0.000000000000   ,  \"στ1\" -> 0.000000000000   ,  \"στS\" -> 0.000000000000   ,  \"στN\" -> 0.000000000000    |>   , \n\"IDS0544_220606_RAW_cal__ref_\" ->   <|    \"ζ\" -> 0.664244638441   ,  \"τ1\" -> 0.246856024037   ,  \"τS\" -> 0.027685516986   ,  \"τN\" -> 0.022864655649   ,  \"τC\" -> 0.000854076829   ,  \"κ0\" -> 0.000000000436   ,  \"mm1\" -> 0.000337098347   ,  \"mm2\" -> 0.039372294078   ,  \"mm3\" -> 0.292128562221   ,  \"T\" -> 0.120000000000   ,  \"B\" -> 2.000000000000   ,  \"θ\" -> 45.000000000000   ,  \"Reoff\" -> -183040816.326530635000   ,  \"Imoff\" -> 0.000000000000   ,  \"στ1\" -> 0.607479321028   ,  \"στS\" -> 0.003421096587   ,  \"στN\" -> 0.047598917320    |>   , \n\"IDS0544_220606_RAW_cal__sam_\" ->   <|    \"ζ\" -> 0.000000000000   ,  \"τ1\" -> 0.000000000000   ,  \"τS\" -> 0.000000000000   ,  \"τN\" -> 0.000000000000   ,  \"τC\" -> 0.000000000000   ,  \"κ0\" -> 0.000000000000   ,  \"mm1\" -> 0.000000000000   ,  \"mm2\" -> 0.000000000000   ,  \"mm3\" -> 0.000000000000   ,  \"T\" -> 0.120000000000   ,  \"B\" -> 2.000000000000   ,  \"θ\" -> 45.000000000000   ,  \"Reoff\" -> 0.000000000000   ,  \"Imoff\" -> 0.000000000000   ,  \"στ1\" -> 0.000000000000   ,  \"στS\" -> 0.000000000000   ,  \"στN\" -> 0.000000000000    |>   , \n\"IDS0545_220606_RAW_cal__ref_\" ->   <|    \"ζ\" -> 0.114584837195   ,  \"τ1\" -> 0.375837377440   ,  \"τS\" -> 0.013356599543   ,  \"τN\" -> 0.007350942831   ,  \"τC\" -> 0.001154352119   ,  \"κ0\" -> 0.000000001547   ,  \"mm1\" -> 0.000110898808   ,  \"mm2\" -> 0.015576445529   ,  \"mm3\" -> 0.384384697967   ,  \"T\" -> 0.300000000000   ,  \"B\" -> 2.000000000000   ,  \"θ\" -> 45.000000000000   ,  \"Reoff\" -> -9836734.693877555430   ,  \"Imoff\" -> 0.000000000000   ,  \"στ1\" -> 0.036231793577   ,  \"στS\" -> 0.000070867254   ,  \"στN\" -> 0.000621210167    |>   , \n\"IDS0545_220606_RAW_cal__sam_\" ->   <|    \"ζ\" -> 0.000000000000   ,  \"τ1\" -> 0.000000000000   ,  \"τS\" -> 0.000000000000   ,  \"τN\" -> 0.000000000000   ,  \"τC\" -> 0.000000000000   ,  \"κ0\" -> 0.000000000000   ,  \"mm1\" -> 0.000000000000   ,  \"mm2\" -> 0.000000000000   ,  \"mm3\" -> 0.000000000000   ,  \"T\" -> 0.300000000000   ,  \"B\" -> 2.000000000000   ,  \"θ\" -> 45.000000000000   ,  \"Reoff\" -> 0.000000000000   ,  \"Imoff\" -> 0.000000000000   ,  \"στ1\" -> 0.000000000000   ,  \"στS\" -> 0.000000000000   ,  \"στN\" -> 0.000000000000    |>   , \n\"IDS0546_220606_RAW_cal__ref_\" ->   <|    \"ζ\" -> 0.086559942010   ,  \"τ1\" -> 0.376689726376   ,  \"τS\" -> 0.013025220586   ,  \"τN\" -> 0.006974345540   ,  \"τC\" -> 0.001217354577   ,  \"κ0\" -> 0.000000001917   ,  \"mm1\" -> 0.000089822592   ,  \"mm2\" -> 0.014966812259   ,  \"mm3\" -> 0.384581173512   ,  \"T\" -> 0.360000000000   ,  \"B\" -> 2.000000000000   ,  \"θ\" -> 45.000000000000   ,  \"Reoff\" -> -8612244.897959187630   ,  \"Imoff\" -> 0.000000000000   ,  \"στ1\" -> 0.438938204284   ,  \"στS\" -> 0.000131885488   ,  \"στN\" -> 0.003309064048    |>   , \n\"IDS0546_220606_RAW_cal__sam_\" ->   <|    \"ζ\" -> 0.000000000000   ,  \"τ1\" -> 0.000000000000   ,  \"τS\" -> 0.000000000000   ,  \"τN\" -> 0.000000000000   ,  \"τC\" -> 0.000000000000   ,  \"κ0\" -> 0.000000000000   ,  \"mm1\" -> 0.000000000000   ,  \"mm2\" -> 0.000000000000   ,  \"mm3\" -> 0.000000000000   ,  \"T\" -> 0.360000000000   ,  \"B\" -> 2.000000000000   ,  \"θ\" -> 45.000000000000   ,  \"Reoff\" -> 0.000000000000   ,  \"Imoff\" -> 0.000000000000   ,  \"στ1\" -> 0.000000000000   ,  \"στS\" -> 0.000000000000   ,  \"στN\" -> 0.000000000000    |>   , \n\"IDS0547_220606_RAW_cal__ref_\" ->   <|    \"ζ\" -> 0.069999106625   ,  \"τ1\" -> 0.375220053416   ,  \"τS\" -> 0.013216291389   ,  \"τN\" -> 0.005647516312   ,  \"τC\" -> 0.001254063929   ,  \"κ0\" -> 0.000000002317   ,  \"mm1\" -> 0.000075729851   ,  \"mm2\" -> 0.015067056915   ,  \"mm3\" -> 0.381515587966   ,  \"T\" -> 0.420000000000   ,  \"B\" -> 2.000000000000   ,  \"θ\" -> 45.000000000000   ,  \"Reoff\" -> -7142857.142857141800   ,  \"Imoff\" -> 0.000000000000   ,  \"στ1\" -> 0.247259195832   ,  \"στS\" -> 0.000163525957   ,  \"στN\" -> 0.005342009137    |>   , \n\"IDS0547_220606_RAW_cal__sam_\" ->   <|    \"ζ\" -> 0.000000000000   ,  \"τ1\" -> 0.000000000000   ,  \"τS\" -> 0.000000000000   ,  \"τN\" -> 0.000000000000   ,  \"τC\" -> 0.000000000000   ,  \"κ0\" -> 0.000000000000   ,  \"mm1\" -> 0.000000000000   ,  \"mm2\" -> 0.000000000000   ,  \"mm3\" -> 0.000000000000   ,  \"T\" -> 0.420000000000   ,  \"B\" -> 2.000000000000   ,  \"θ\" -> 45.000000000000   ,  \"Reoff\" -> 0.000000000000   ,  \"Imoff\" -> 0.000000000000   ,  \"στ1\" -> 0.000000000000   ,  \"στS\" -> 0.000000000000   ,  \"στN\" -> 0.000000000000    |>   , \n\"IDS0548_220606_RAW_cal__ref_\" ->   <|    \"ζ\" -> 0.050401769736   ,  \"τ1\" -> 0.373876419184   ,  \"τS\" -> 0.013977187329   ,  \"τN\" -> 0.005482355270   ,  \"τC\" -> 0.001501801590   ,  \"κ0\" -> 0.000000002989   ,  \"mm1\" -> 0.000065640074   ,  \"mm2\" -> 0.015862773261   ,  \"mm3\" -> 0.379890145424   ,  \"T\" -> 0.520000000000   ,  \"B\" -> 2.000000000000   ,  \"θ\" -> 45.000000000000   ,  \"Reoff\" -> -3714285.714285716420   ,  \"Imoff\" -> 0.000000000000   ,  \"στ1\" -> 0.110713266907   ,  \"στS\" -> 0.000122907745   ,  \"στN\" -> 0.001966965268    |>   , \n\"IDS0548_220606_RAW_cal__sam_\" ->   <|    \"ζ\" -> 0.000000000000   ,  \"τ1\" -> 0.000000000000   ,  \"τS\" -> 0.000000000000   ,  \"τN\" -> 0.000000000000   ,  \"τC\" -> 0.000000000000   ,  \"κ0\" -> 0.000000000000   ,  \"mm1\" -> 0.000000000000   ,  \"mm2\" -> 0.000000000000   ,  \"mm3\" -> 0.000000000000   ,  \"T\" -> 0.520000000000   ,  \"B\" -> 2.000000000000   ,  \"θ\" -> 45.000000000000   ,  \"Reoff\" -> 0.000000000000   ,  \"Imoff\" -> 0.000000000000   ,  \"στ1\" -> 0.000000000000   ,  \"στS\" -> 0.000000000000   ,  \"στN\" -> 0.000000000000    |>   , \n\"IDS0549_220606_RAW_cal__ref_\" ->   <|    \"ζ\" -> 0.041979401075   ,  \"τ1\" -> 0.368478793966   ,  \"τS\" -> 0.015446799439   ,  \"τN\" -> 0.003402337716   ,  \"τC\" -> 0.001575093876   ,  \"κ0\" -> 0.000000003686   ,  \"mm1\" -> 0.000057991267   ,  \"mm2\" -> 0.017436315900   ,  \"mm3\" -> 0.372199993318   ,  \"T\" -> 0.620000000000   ,  \"B\"
